vi "main.vi"() -> ()   [LabVIEW 2013]
uses:
  <vilib>/NXT/NXT Controls/ConnectionType.ctl
  <vilib>/NXT/Block Support/NXT_InputPort.ctl
  <vilib>/NXT/Block Support/HWPage.SensorType.ctl
  <vilib>/NXT/Block Support/HWPage.SensorMode.ctl
  <vilib>/NXT/Block Support/NXT_OutputPort.ctl
  <vilib>/Utility/inputDevices.llb/closeJoystick.vi
  <vilib>/NXT/Dual Mode Library/Sensors/i2c_sensors_big.vi
  <vilib>/NXT/Dual Mode Library/Sensors/Sonar_cm.vi
  <vilib>/NXT/Dual Mode Library/Sensors/EV3_Infrared_Proxy.vi
  <vilib>/NXT/Dual Mode Library/Sensors/Read_Battery.vi
  <vilib>/Utility/inputDevices.llb/joystickAcquire.vi
  <vilib>/NXT/NXTIO Xnodes/NXTIONodeSubVIs/NXTMoveMotors.vi
  <vilib>/NXT/Dual Mode Library/Sound/Tone.vi
  <vilib>/NXT/NXTIO Xnodes/NXTIONodeSubVIs/NXTStopMotors.vi
  <vilib>/NXT/NXTIO Xnodes/AddressXNode/NXTIOAddress.xnode
  <vilib>/NXT/NXTIO Xnodes/NXTIOXNode/NXTIO.xnode
  <vilib>/NXT/Subs/LVHSConnector.ctl
  <vilib>/NXT/LegoClasses/BrickReference/BrickReference.lvclass
panel:
  out "Distance - right":i32
  out "Distance - left":i32
  in  "Arduino port":T1 items=["Port 1", "Port 2", "Port 3", "Port 4"]
  in  "Aft sensor port":T1 items=["Port 1", "Port 2", "Port 3", "Port 4"]
  in  "Front sensor port":T1=3 items=["Port 1", "Port 2", "Port 3", "Port 4"]
  in  "Connection Type":T2=enum."USB"
  in  "NXT/EV3 name":string
  out "Distance - Front":i16
  out "Distance - Aft":sgl
  out "Voltage":dbl
  in  "Enable throttle":bool
  out "Battery voltage [V]":sgl(slide) scale=0.0..10.0
  in  "Stop Button":bool
  out "throttle":dbl(knob) scale=0.0..100.0
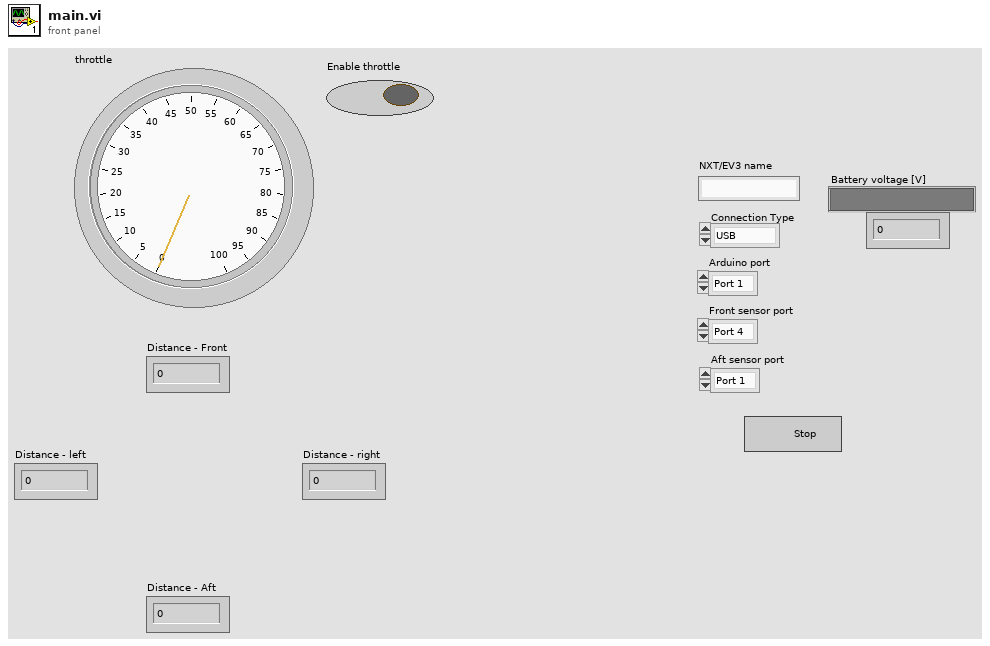
[diagram p1: front panel]
types:
  T1 = typedef "NXT_InputPort.ctl" = u32
  T2 = typedef "ConnectionType.ctl" = enum16{"Bluetooth", "USB", "WiFi"}
  T3 = typedef "HWPage.SensorType.ctl" = u8
  T4 = typedef "HWPage.SensorMode.ctl" = u8
  T5 = typedef "LVHSConnector.ctl" = refnum<class "BrickReference.lvclass">
  T6 = typedef "NXT_OutputPort.ctl" = u8
  T7 = cluster{"X axis":i32, "Y axis":i32, "Z axis":i32, "X axis rotation":i32, "Y axis rotation":i32, "Z axis rotation":i32, "U axis":i32, "V axis":i32}
  T8 = cluster{"X axis":dbl, "Y axis":dbl, "Z axis":dbl, "X axis rotation":dbl, "Y axis rotation":dbl, "Z axis rotation":dbl, "U axis":dbl, "V axis":dbl}
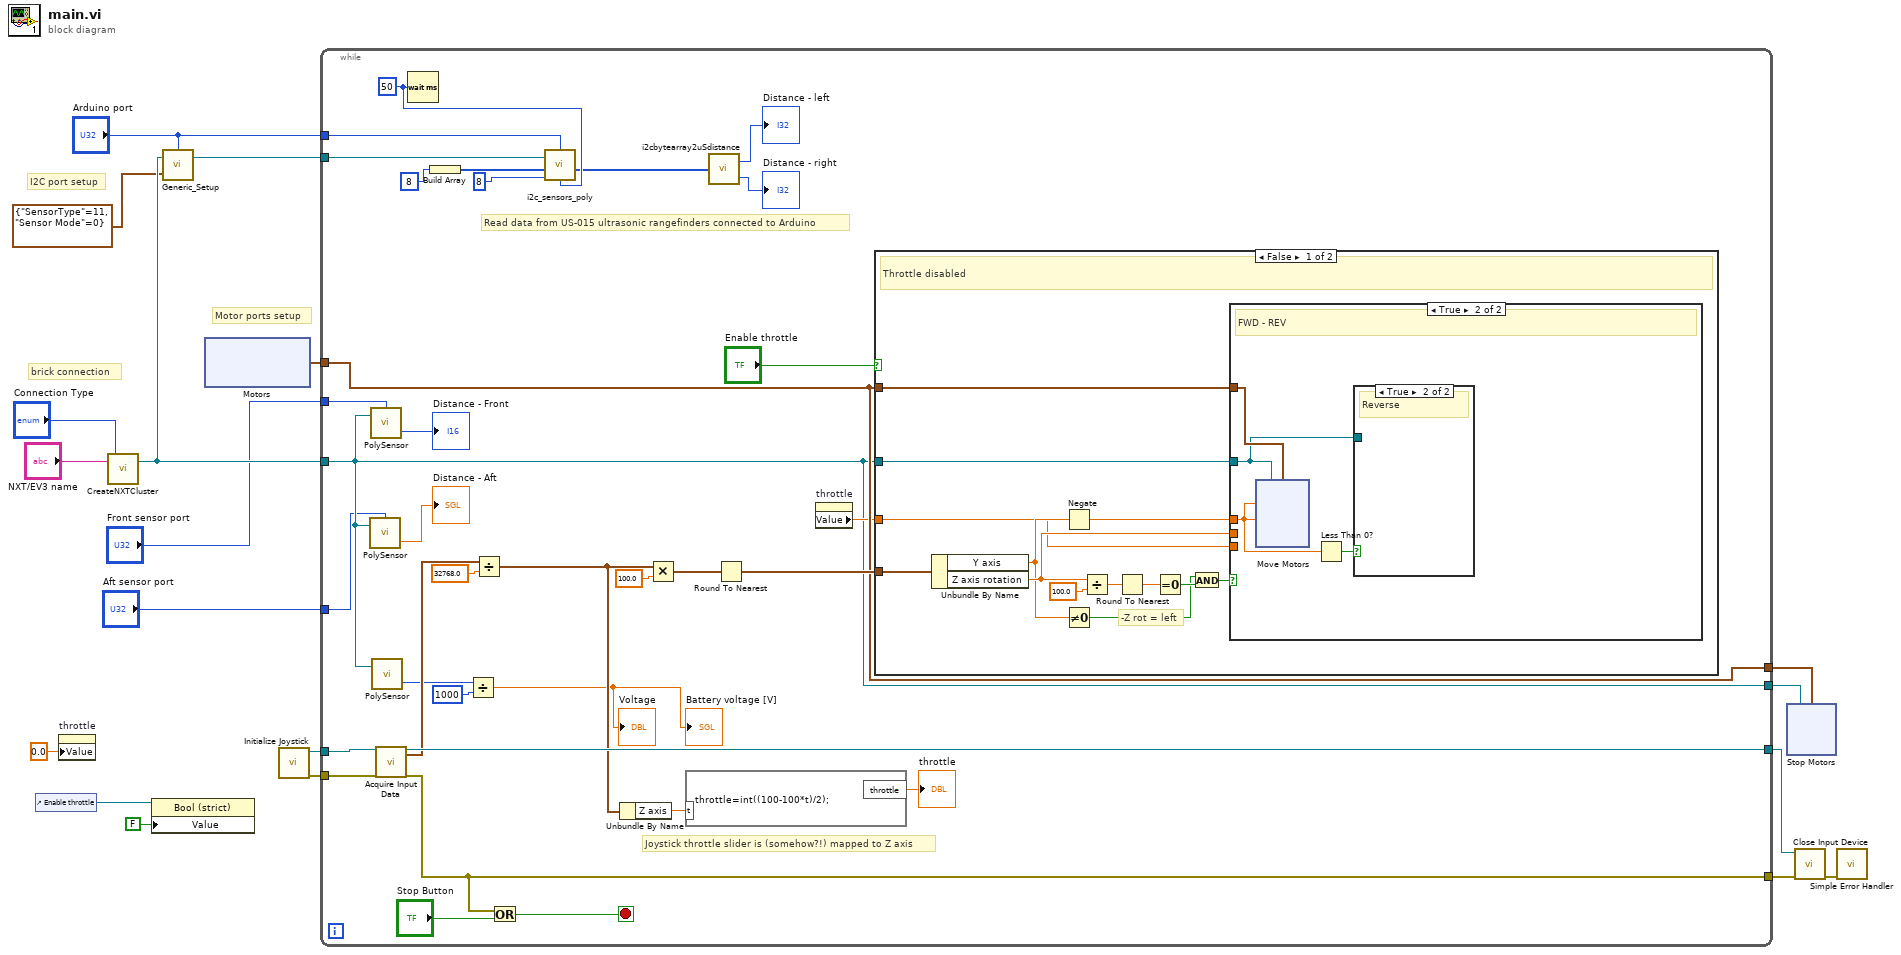
[diagram p0: block diagram]
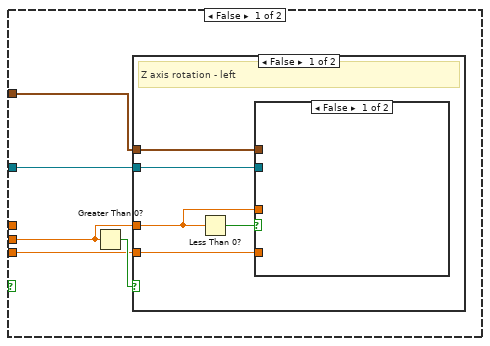
[diagram p2: hidden frame]
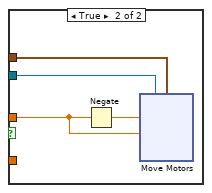
[diagram p3: hidden frame]
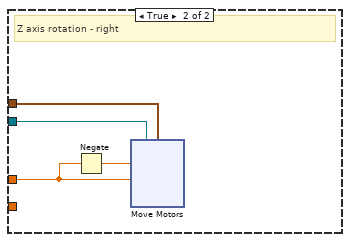
[diagram p4: hidden frame]
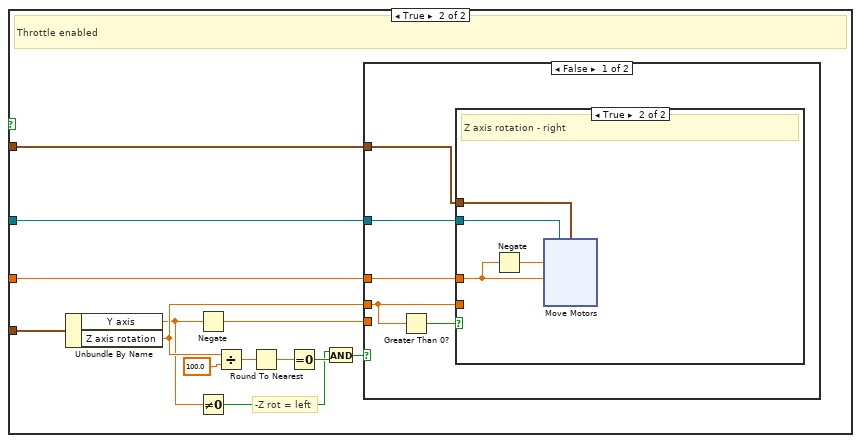
[diagram p6: hidden frame]
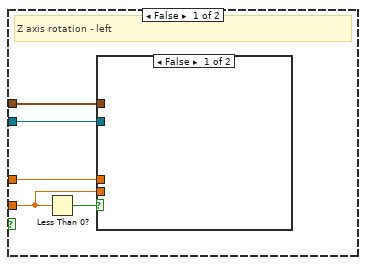
[diagram p7: hidden frame]
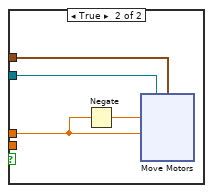
[diagram p8: hidden frame]
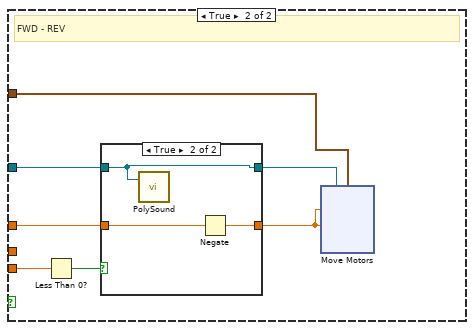
[diagram p9: hidden frame]
diagram:
  # "Motor ports setup"
  # "brick connection"
  # "I2C port setup"
  n1 = control-ref of="Enable throttle"() -> (w10:refnum<vi>)
  n2 = property on="throttle" class="Knob (strict)"("Value"=0.0 ("throttle")) -> ()  [unwired: 2 in, 2 out]
  n3 = call <vilib>:"CreateNXTCluster.vi"("Connection Type"="Connection Type", "NXT/EV3 name"="NXT/EV3 name") -> ("NXT/EV3"=w7:T5)  [unwired: 2 in]
  n4 = property class="Bool (strict)"(reference=w10, "Value"=FALSE) -> ()  [unwired: 1 in, 2 out]
  n5 = call <vilib>:"Generic_Setup.vi"("Sensor Setup"=cluster{"SensorType":T3, "Sensor Mode":T4} {"SensorType"=11, "Sensor Mode"=0}, "NXT/EV3"=w7, "Port"="Arduino port") -> ("NXT/EV3"=w5:T5)  [unwired: 1 out]
  n6 = xnode "Motors"() -> ("Motor"=w11:cluster{"Port":T6, "Port":T6})
  n7 = call <vilib>:"Initialize Joystick.vi"() -> ("error out"=w18:errorcluster, "device ID"=w19:refnum<k1>)  [unwired: 10 in]
  n8 = while {
    tunnel: w19 -> [w53]
    tunnel: w18 -> [w52]
    tunnel: [w49] -> w17
    tunnel: [w51] -> w16
    tunnel: w7 -> [w29]
    tunnel: [w29] -> w13
    tunnel: [w35] -> w12
    tunnel: w11 -> [w35]
    tunnel: w5 -> [w33]
    tunnel: "Arduino port" -> [w26]
    tunnel: "Front sensor port" -> [w25]
    tunnel: "Aft sensor port" -> [w24]
    stop <- w50 stop-if-true
    w23 = u32 50 ("milliseconds to wait")
    # "Joystick throttle slider is (somehow?!) mapped to Z axis"
    # "Read data from US-015 ultrasonic rangefinders connected to Arduino"
    n9 = call-poly <vilib>:"PolySensor.vi"("NXT/EV3"=w29, "Port (Port 1)"=w24) -> ("Scaled Value"=→"Distance - Aft":sgl)  [unwired: 1 in, 1 out]
    n10 = call-poly <vilib>:"PolySensor.vi"("NXT/EV3"=w29, "Port (Port 4)"=w25) -> ("Distance (cm)"=→"Distance - Front":i16)  [unwired: 1 in, 1 out]
    n11 = call-poly <vilib>:"PolySensor.vi"("NXT/EV3"=w29) -> ("millivolts"=w38:i32)  [unwired: 2 in, 1 out]
    n12 = call-poly <vilib>:"Acquire Input Data.vi"("device ID"=w53, "error in (no error)"=w52) -> ("device ID"=w51:refnum<k1>, "axis info"=w47:T7, "error out"=w49:errorcluster)  [unwired: 13 in, 2 out]
    n13 = Wait (ms)(milliseconds to wait=w23) -> ()  [unwired: 1 out]
    n14 = Build Array(8) -> (w30:i32[])
    n15 = Divide(x=w38, y=1000) -> (x/y=→"Battery voltage [V]" →"Voltage":dbl)
    n16 = Divide(x=w47, y=32768.0) -> (x/y=w43:T8)
    n17 = Or(x=w49, y="Stop Button") -> (x .or. y?=w50:bool)
    n18 = call-poly <vilib>:"i2c_sensors_poly.vi"("Return Length"=u8 8, "Bytes to Write"=w30, "Wait (msec)"=w23, "NXT/EV3"=w33, "Port"=w26) -> ("Bytes read"=w22:u8[])  [unwired: 2 out]
    n19 = Unbundle By Name(w43) -> ("Z axis"=w45:dbl)
    n20 = Multiply(x=w43, y=100.0) -> (x*y=w42:T8)
    n21 = formula code="throttle=int((100-100*t)/2);"("t"=w45) -> ("throttle"=→"throttle":dbl)
    n22 = call "i2cbytearray2uSdistance.vi"("Bytes read"=w22) -> ("Distance - left"=→"Distance - left":i32, "Distance - right"=→"Distance - right":i32)
    n23 = Round To Nearest(number=w42) -> (nearest integer value=w39:T8)
    n24 = property on="throttle" class="Knob (strict)"() -> ("Value"=w34:dbl)  [unwired: 2 in, 2 out]
    n25 = case shown="False" "Enable throttle" {
      tunnel: w29 -> [w65 w116]
      tunnel: w39 -> [w66 w115]
      tunnel: w35 -> [w64 w114]
      tunnel: w34 -> [w54 w113]
      frame False {
        # "-Z rot = left"
        # "Throttle disabled"
        n26 = Unbundle By Name(w66) -> ("Y axis"=w56:dbl, "Z axis rotation"=w60:dbl)
        n27 = Negate(x=w56) -> (-x=w55:dbl)
        n28 = Not Equal To 0?(x=w56) -> (x != 0?=w61:bool)
        n29 = Divide(x=w60, y=100.0) -> (x/y=w58:dbl)
        n30 = Round To Nearest(number=w58) -> (nearest integer value=w57:dbl)
        n31 = Equal To 0?(x=w57) -> (x = 0?=w63:bool)
        n32 = And(x=w61, y=w63) -> (x .and. y?=w62:bool)
        n33 = case shown="True" w62 {
          tunnel: w65 -> [w69 w101]
          tunnel: w64 -> [w70 w104]
          tunnel: w55 -> [_ w103]
          tunnel: w60 -> [w68 _]
          tunnel: w54 -> [w67 _]
          frame False {
            n34 = Greater Than 0?(x=w68) -> (x > 0?=w71:bool)
            n35 = case shown="False" w71 {
              tunnel: w70 -> [w74 w92]
              tunnel: w69 -> [w75 w91]
              tunnel: w68 -> [w73 w89]
              tunnel: w67 -> [w72 _]
              frame False {
                # "Z axis rotation - left"
                n36 = Less Than 0?(x=w73) -> (x < 0?=w76:bool)
                n37 = case shown="False" w76 {
                  tunnel: w75 -> [_ w80]
                  tunnel: w74 -> [_ w79]
                  tunnel: w73 -> [_ w77]
                  tunnel: w72 -> [_ _]
                  frame False {
                  }
                  frame True {
                    n38 = Negate(x=w77) -> (-x=w78:dbl)
                    n39 = xnode "Move Motors"("Power/Speed 2"=w77, "Power/Speed 1"=w78, "Motors"=w79, "NXT/EV3"=w80) -> ()  [unwired: 1 out]
                  }
                }
              }
              frame True {
                # "Z axis rotation - right"
                n40 = Negate(x=w89) -> (-x=w90:dbl)
                n41 = xnode "Move Motors"("Power/Speed 2"=w89, "Power/Speed 1"=w90, "Motors"=w92, "NXT/EV3"=w91) -> ()  [unwired: 1 out]
              }
            }
          }
          frame True {
            # "FWD - REV"
            n42 = xnode "Move Motors"("Power/Speed 2"=w103, "Power/Speed 1"=w103, "Motors"=w104, "NXT/EV3"=w101) -> ()  [unwired: 1 out]
            n43 = Less Than 0?(x=w103) -> (x < 0?=w102:bool)
            n44 = case shown="True" w102 {
              tunnel: w101 -> [_ _]
              frame False {
              }
              frame True {
                # "Reverse"
              }
            }
          }
        }
      }
      frame True {
        # "-Z rot = left"
        # "Throttle enabled"
        n45 = Unbundle By Name(w115) -> ("Y axis"=w118:dbl, "Z axis rotation"=w122:dbl)
        n46 = Negate(x=w118) -> (-x=w117:dbl)
        n47 = Not Equal To 0?(x=w118) -> (x != 0?=w123:bool)
        n48 = Divide(x=w122, y=100.0) -> (x/y=w120:dbl)
        n49 = Round To Nearest(number=w120) -> (nearest integer value=w119:dbl)
        n50 = Equal To 0?(x=w119) -> (x = 0?=w125:bool)
        n51 = And(x=w123, y=w125) -> (x .and. y?=w124:bool)
        n52 = case shown="False" w124 {
          tunnel: w116 -> [w128 w164]
          tunnel: w114 -> [w129 w161]
          tunnel: w117 -> [_ w166]
          tunnel: w122 -> [w127 _]
          tunnel: w113 -> [w126 w162]
          frame False {
            n53 = Greater Than 0?(x=w127) -> (x > 0?=w130:bool)
            n54 = case shown="True" w130 {
              tunnel: w129 -> [w133 w151]
              tunnel: w128 -> [w134 w150]
              tunnel: w127 -> [w132 _]
              tunnel: w126 -> [w131 w148]
              frame False {
                # "Z axis rotation - left"
                n55 = Less Than 0?(x=w132) -> (x < 0?=w135:bool)
                n56 = case shown="False" w135 {
                  tunnel: w134 -> [_ w139]
                  tunnel: w133 -> [_ w138]
                  tunnel: w132 -> [_ _]
                  tunnel: w131 -> [_ w136]
                  frame False {
                  }
                  frame True {
                    n57 = Negate(x=w136) -> (-x=w137:dbl)
                    n58 = xnode "Move Motors"("Power/Speed 2"=w136, "Power/Speed 1"=w137, "Motors"=w138, "NXT/EV3"=w139) -> ()  [unwired: 1 out]
                  }
                }
              }
              frame True {
                # "Z axis rotation - right"
                n59 = Negate(x=w148) -> (-x=w149:dbl)
                n60 = xnode "Move Motors"("Power/Speed 2"=w148, "Power/Speed 1"=w149, "Motors"=w151, "NXT/EV3"=w150) -> ()  [unwired: 1 out]
              }
            }
          }
          frame True {
            # "FWD - REV"
            n61 = Less Than 0?(x=w166) -> (x < 0?=w165:bool)
            n62 = case shown="True" w165 {
              tunnel: w164 -> [w167 w171]
              tunnel: [w167 w171] -> w163
              tunnel: w162 -> [w168 w170]
              tunnel: [w168 w169] -> w160
              frame False {
              }
              frame True {
                n63 = call-poly <vilib>:"PolySound.vi"("NXT/EV3"=w171) -> ()  [unwired: 3 in, 1 out]
                n64 = Negate(x=w170) -> (-x=w169:dbl)
              }
            }
            n65 = xnode "Move Motors"("Power/Speed 2"=w160, "Power/Speed 1"=w160, "Motors"=w161, "NXT/EV3"=w163) -> ()  [unwired: 1 out]
          }
        }
      }
    }
  }
  n66 = xnode "Stop Motors"("Motors"=w12, "NXT/EV3"=w13) -> ()  [unwired: 1 out]
  n67 = call-poly <vilib>:"Close Input Device.vi"("error in (no error)"=w17, "device ID"=w16) -> ("error out"=w4:errorcluster)  [unwired: 8 in]
  n68 = call <vilib>:"Simple Error Handler.vi"("error in (no error)"=w4) -> ()  [unwired: 4 in, 5 out]
